vi "read product name.vi"(11 "Builders in":refnum<class "Builder.lvclass">) -> (2 "product name":string)   [LabVIEW 2024, in "Builder.lvclass"]
uses:
  Builder.lvclass
  Builder.lvclass/Builder.ctl
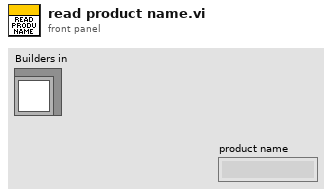
[diagram p1: front panel]
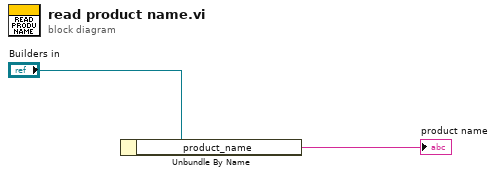
[diagram p0: block diagram]
diagram:
  n1 = Unbundle By Name("Builders in") -> ("product_name"=→"product name":string)
